vi "Write Hallway.vi"(8 "error in (no error)":errorcluster, 10 "Hallway":string[](array[string]), 11 "State Key in":refnum<class "State Key.lvclass">) -> (0 "error out":errorcluster, 3 "State Key out":refnum<class "State Key.lvclass">)   [LabVIEW 2019, in "23.lvlib" / "State Key.lvclass"]
uses:
  State Key.lvclass
  State Key.lvclass/State Key.ctl
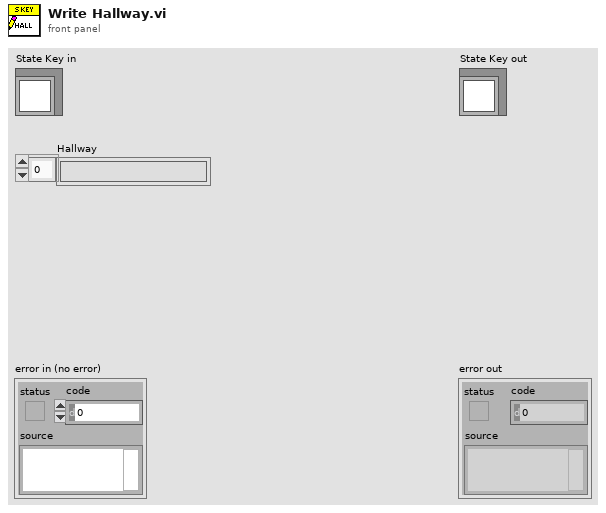
[diagram p1: front panel]
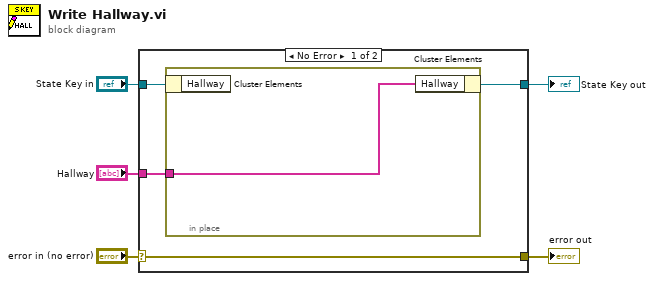
[diagram p0: block diagram]
diagram:
  n1 = case shown="No Error" "error in (no error)" {
    selector: "error in (no error)" -> [w9 w11]
    tunnel: [w9 w11] -> w4
    tunnel: [w6 w12] -> w2
    tunnel: "State Key in" -> [w7 w12]
    tunnel: "Hallway" -> [w8 _]
    frame No Error {
      n2 = in-place {
        in-place-border: w8 -> [w10]
        n3 = in-place-cluster #1(w7) -> ()  [unwired: 1 out]
        n4 = in-place-cluster #1("Hallway"=w10) -> (w6:refnum<class "State Key.lvclass">)
      }
    }
    frame Error {
    }
  }
  "error out" <- w4
  "State Key out" <- w2
